vi "WILT Increment Cycle.vi"(5 "Station Number in":u32, 6 "Short Cycle?":bool, 7 "Day/Night Cycle":T7, 8 "Error In":errorcluster, 10 "Station Test State In":T1, 11 "Dryer Step 5 In":T3 {"Night Cycle Count" format="%04d"; "Day Cycle Count" format="%04d"}) -> (0 "Error Out":errorcluster, 1 "Enable Start Retry":bool, 2 "Test Station Out":T1, 3 "Dryer Step 5 Output":T3 {"Night Cycle Count" format="%04d"; "Day Cycle Count" format="%04d"})   [LabVIEW 2016]
uses:
  Type Definitions/WILT Day Night Cycle Enum.ctl
  Type Definitions/WILT Dryer.ctl
  Type Definitions/WILT Dryer Details.ctl
  Type Definitions/WILT Agilent Channel Definition.ctl
  Type Definitions/WILT DAQ Data.ctl
  Type Definitions/WILT Station Test State Cluster.ctl
  Type Definitions/WILT Dryer Test State.ctl
panel:
  # "Day"
  # "Night"
  # "Day"
  # "Night"
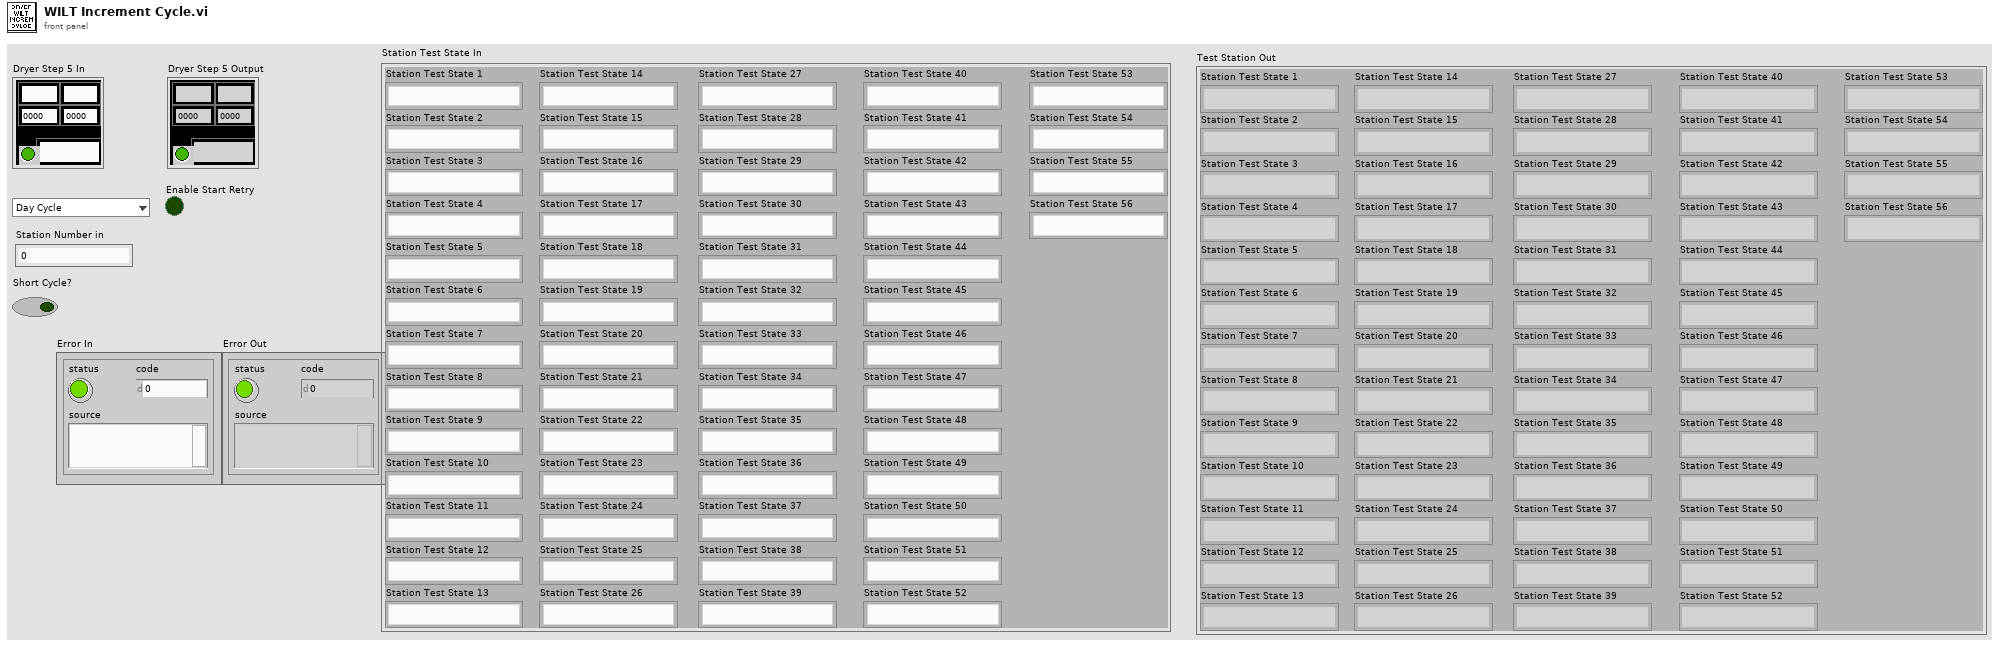
[diagram p1: front panel]
types:
  T1 = typedef "WILT Station Test State Cluster.ctl" = cluster{"Station Test State 1":T2, "Station Test State 2":T2, "Station Test State 3":T2, "Station Test State 4":T2, "Station Test State 5":T2, "Station Test State 6":T2, "Station Test State 7":T2, "Station Test State 8":T2, "Station Test State 9":T2, "Station Test State 10":T2, "Station Test State 11":T2, "Station Test State 12":T2, "Station Test State 13":T2, "Station Test State 14":T2, "Station Test State 15":T2, "Station Test State 16":T2, "Station Test State 17":T2, "Station Test State 18":T2, "Station Test State 19":T2, "Station Test State 20":T2, "Station Test State 21":T2, "Station Test State 22":T2, "Station Test State 23":T2, "Station Test State 24":T2, "Station Test State 25":T2, "Station Test State 26":T2, "Station Test State 27":T2, "Station Test State 28":T2, "Station Test State 29":T2, "Station Test State 30":T2, "Station Test State 31":T2, "Station Test State 32":T2, "Station Test State 33":T2, "Station Test State 34":T2, "Station Test State 35":T2, "Station Test State 36":T2, "Station Test State 37":T2, "Station Test State 38":T2, "Station Test State 39":T2, "Station Test State 40":T2, "Station Test State 41":T2, "Station Test State 42":T2, "Station Test State 43":T2, "Station Test State 44":T2, "Station Test State 45":T2, "Station Test State 46":T2, "Station Test State 47":T2, "Station Test State 48":T2, "Station Test State 49":T2, "Station Test State 50":T2, "Station Test State 51":T2, "Station Test State 52":T2, "Station Test State 53":T2, "Station Test State 54":T2, "Station Test State 55":T2, "Station Test State 56":T2}
  T2 = typedef "WILT Dryer Test State.ctl" = enum16{"No Serial Number", "Waiting for Dryer To Start", "Drying Clothes", "Water Injection 1 (On)", "Water Injection 1 Timer", "Water Injection 1 (Off)", "Pause Dryer", "Sending Start Stop CMD", "Pause Dryer 2", "Sending Start Stop CMD 2", "Drying Clothes 2", "Water Injection 2 (On)", "Water Injection 2 Timer", "Water Injection 2 (Off)", "Drying Clothes 3", "Cooling Down", "Sending Start Stop CMD 3", "Increment Cycle"}
  T3 = typedef "WILT Dryer.ctl" = cluster{"Lab ID":string, "Day Cycle Count":i32, "Station Label":string, "Dryer Details":T4, "Status Color":u32, "Invisible Button":bool, "Night Cycle Count":i32, "Station Index":i32, "Cycle Index":string, "Audit Alert":bool, "Agilent Channel Definition":T5, "DAQ Data":T6}
  T4 = typedef "WILT Dryer Details.ctl" = cluster{"Station":string, "Lab ID":string, "TR Number":string}
  T5 = typedef "WILT Agilent Channel Definition.ctl" = cluster{"Channel":string, "Station":string, "Label":string, "Agilent Station":string, "Data":dbl}
  T6 = typedef "WILT DAQ Data.ctl" = cluster{"L1 Current":dbl, "L2 Current":dbl, "Temperature  Deg F (TC)":dbl, "Volts":dbl, "Volts (208)":dbl, "SW (208)":dbl}
  T7 = typedef "WILT Day Night Cycle Enum.ctl" = enum16{"Day Cycle", "Night Cycle", "Day Cycle (No Water)"}
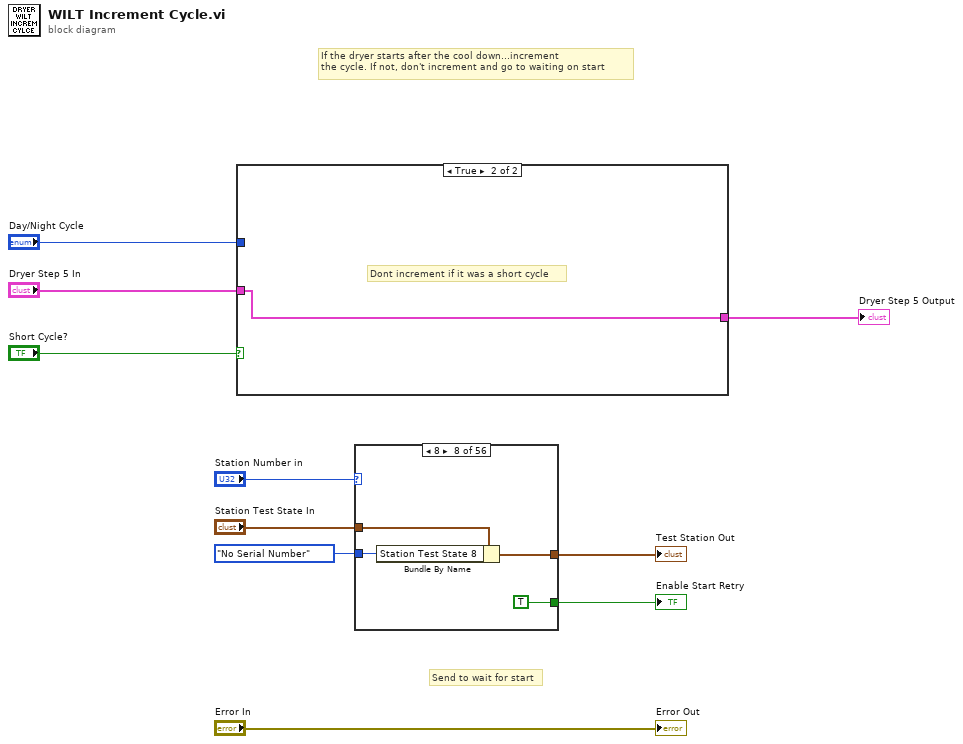
[diagram p0: block diagram]
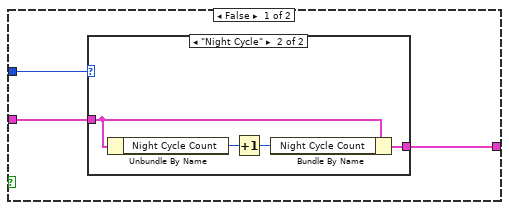
[diagram p2: hidden frame]
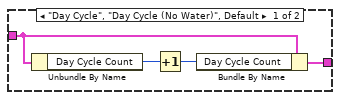
[diagram p3: hidden frame]
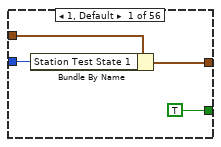
[diagram p4: hidden frame]
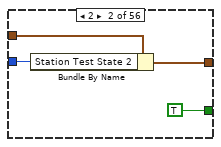
[diagram p5: hidden frame]
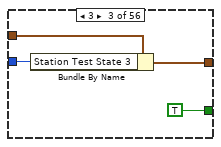
[diagram p6: hidden frame]
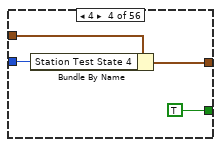
[diagram p7: hidden frame]
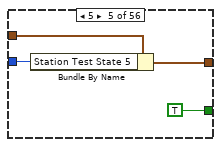
[diagram p8: hidden frame]
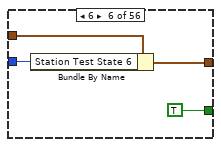
[diagram p9: hidden frame]
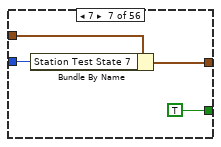
[diagram p10: hidden frame]
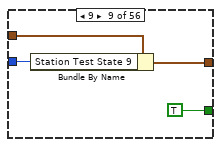
[diagram p11: hidden frame]
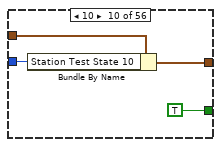
[diagram p12: hidden frame]
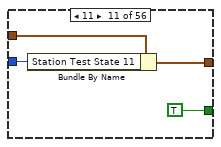
[diagram p13: hidden frame]
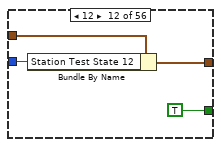
[diagram p14: hidden frame]
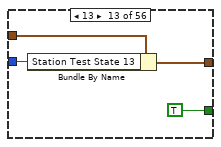
[diagram p15: hidden frame]
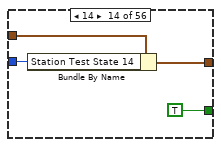
[diagram p16: hidden frame]
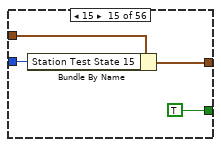
[diagram p17: hidden frame]
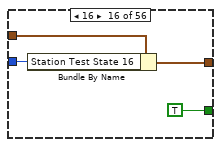
[diagram p18: hidden frame]
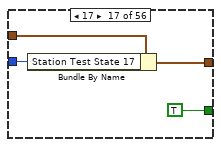
[diagram p19: hidden frame]
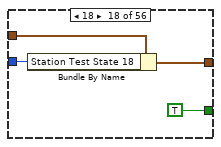
[diagram p20: hidden frame]
diagram:
  # "Send to wait for start"
  # "If the dryer starts after the cool down...increment\nthe cycle. If not, don't increment and go to waiting on start"
  n1 = case shown="True" "Short Cycle?" {
    tunnel: "Day/Night Cycle" -> [w13 _]
    tunnel: [w12 w22] -> w8
    tunnel: "Dryer Step 5 In" -> [w11 w22]
    frame False {
      n2 = case shown="\"Night Cycle\"" w13 {
        tunnel: w11 -> [w14 w18]
        tunnel: [w17 w21] -> w12
        frame "Day Cycle", "Day Cycle (No Water)", Default {
          n3 = Unbundle By Name(w14) -> ("Day Cycle Count"=w16:i32)
          n4 = Increment(x=w16) -> (x+1=w15:i32)
          n5 = Bundle By Name(cluster=w14, "Day Cycle Count"=w15) -> (w17:T3)
        }
        frame "Night Cycle" {
          n6 = Unbundle By Name(w18) -> ("Night Cycle Count"=w20:i32)
          n7 = Increment(x=w20) -> (x+1=w19:i32)
          n8 = Bundle By Name(cluster=w18, "Night Cycle Count"=w19) -> (w21:T3)
        }
      }
    }
    frame True {
      # "Dont increment if it was a short cycle"
    }
  }
  "Dryer Step 5 Output" <- w8
  n9 = case shown="8" "Station Number in" {
    tunnel: "Station Test State In" -> [w26 w30 w34 w38 w42 w46 w50 w54 w58 w62 w66 w70 w74 w78 w82 w86 w90 w94 w98 w102 w106 w110 w114 w118 w122 w126 w130 w134 w138 w142 w146 w150 w154 w158 w162 w166 w170 w174 w178 w182 w186 w190 w194 w198 w202 w206 w210 w214 w218 w222 w226 w230 w234 w238 w242 w246]
    tunnel: WILT_Dryer_Test_State."No Serial Number" ("Station Test State 56") -> [w25 w28 w32 w36 w40 w44 w48 w52 w56 w60 w64 w68 w72 w76 w80 w84 w88 w92 w96 w100 w104 w108 w112 w116 w120 w124 w128 w132 w136 w140 w144 w148 w152 w156 w160 w164 w168 w172 w176 w180 w184 w188 w192 w196 w200 w204 w208 w212 w216 w220 w224 w228 w232 w236 w240 w244]
    tunnel: [w24 w29 w33 w37 w41 w45 w49 w53 w57 w61 w65 w69 w73 w77 w81 w85 w89 w93 w97 w101 w105 w109 w113 w117 w121 w125 w129 w133 w137 w141 w145 w149 w153 w157 w161 w165 w169 w173 w177 w181 w185 w189 w193 w197 w201 w205 w209 w213 w217 w221 w225 w229 w233 w237 w241 w245] -> w5
    tunnel: [TRUE TRUE TRUE TRUE TRUE TRUE TRUE TRUE TRUE TRUE TRUE TRUE TRUE TRUE TRUE TRUE TRUE TRUE TRUE TRUE TRUE TRUE TRUE TRUE TRUE TRUE TRUE TRUE TRUE TRUE TRUE TRUE TRUE TRUE TRUE TRUE TRUE TRUE TRUE TRUE TRUE TRUE TRUE TRUE TRUE TRUE TRUE TRUE TRUE TRUE TRUE TRUE TRUE TRUE TRUE TRUE] -> w2
    frame 1, Default {
      n10 = Bundle By Name(cluster=w26, "Station Test State 1"=w25) -> (w24:T1)
    }
    frame 2 {
      n11 = Bundle By Name(cluster=w30, "Station Test State 2"=w28) -> (w29:T1)
    }
    frame 3 {
      n12 = Bundle By Name(cluster=w34, "Station Test State 3"=w32) -> (w33:T1)
    }
    frame 4 {
      n13 = Bundle By Name(cluster=w38, "Station Test State 4"=w36) -> (w37:T1)
    }
    frame 5 {
      n14 = Bundle By Name(cluster=w42, "Station Test State 5"=w40) -> (w41:T1)
    }
    frame 6 {
      n15 = Bundle By Name(cluster=w46, "Station Test State 6"=w44) -> (w45:T1)
    }
    frame 7 {
      n16 = Bundle By Name(cluster=w50, "Station Test State 7"=w48) -> (w49:T1)
    }
    frame 8 {
      n17 = Bundle By Name(cluster=w54, "Station Test State 8"=w52) -> (w53:T1)
    }
    frame 9 {
      n18 = Bundle By Name(cluster=w58, "Station Test State 9"=w56) -> (w57:T1)
    }
    frame 10 {
      n19 = Bundle By Name(cluster=w62, "Station Test State 10"=w60) -> (w61:T1)
    }
    frame 11 {
      n20 = Bundle By Name(cluster=w66, "Station Test State 11"=w64) -> (w65:T1)
    }
    frame 12 {
      n21 = Bundle By Name(cluster=w70, "Station Test State 12"=w68) -> (w69:T1)
    }
    frame 13 {
      n22 = Bundle By Name(cluster=w74, "Station Test State 13"=w72) -> (w73:T1)
    }
    frame 14 {
      n23 = Bundle By Name(cluster=w78, "Station Test State 14"=w76) -> (w77:T1)
    }
    frame 15 {
      n24 = Bundle By Name(cluster=w82, "Station Test State 15"=w80) -> (w81:T1)
    }
    frame 16 {
      n25 = Bundle By Name(cluster=w86, "Station Test State 16"=w84) -> (w85:T1)
    }
    frame 17 {
      n26 = Bundle By Name(cluster=w90, "Station Test State 17"=w88) -> (w89:T1)
    }
    frame 18 {
      n27 = Bundle By Name(cluster=w94, "Station Test State 18"=w92) -> (w93:T1)
    }
    frame 19 {
      n28 = Bundle By Name(cluster=w98, "Station Test State 19"=w96) -> (w97:T1)
    }
    frame 20 {
      n29 = Bundle By Name(cluster=w102, "Station Test State 20"=w100) -> (w101:T1)
    }
    frame 21 {
      n30 = Bundle By Name(cluster=w106, "Station Test State 21"=w104) -> (w105:T1)
    }
    frame 22 {
      n31 = Bundle By Name(cluster=w110, "Station Test State 22"=w108) -> (w109:T1)
    }
    frame 23 {
      n32 = Bundle By Name(cluster=w114, "Station Test State 23"=w112) -> (w113:T1)
    }
    frame 24 {
      n33 = Bundle By Name(cluster=w118, "Station Test State 24"=w116) -> (w117:T1)
    }
    frame 25 {
      n34 = Bundle By Name(cluster=w122, "Station Test State 25"=w120) -> (w121:T1)
    }
    frame 26 {
      n35 = Bundle By Name(cluster=w126, "Station Test State 26"=w124) -> (w125:T1)
    }
    frame 27 {
      n36 = Bundle By Name(cluster=w130, "Station Test State 27"=w128) -> (w129:T1)
    }
    frame 28 {
      n37 = Bundle By Name(cluster=w134, "Station Test State 28"=w132) -> (w133:T1)
    }
    frame 29 {
      n38 = Bundle By Name(cluster=w138, "Station Test State 29"=w136) -> (w137:T1)
    }
    frame 30 {
      n39 = Bundle By Name(cluster=w142, "Station Test State 30"=w140) -> (w141:T1)
    }
    frame 31 {
      n40 = Bundle By Name(cluster=w146, "Station Test State 31"=w144) -> (w145:T1)
    }
    frame 32 {
      n41 = Bundle By Name(cluster=w150, "Station Test State 32"=w148) -> (w149:T1)
    }
    frame 33 {
      n42 = Bundle By Name(cluster=w154, "Station Test State 33"=w152) -> (w153:T1)
    }
    frame 34 {
      n43 = Bundle By Name(cluster=w158, "Station Test State 34"=w156) -> (w157:T1)
    }
    frame 35 {
      n44 = Bundle By Name(cluster=w162, "Station Test State 35"=w160) -> (w161:T1)
    }
    frame 36 {
      n45 = Bundle By Name(cluster=w166, "Station Test State 36"=w164) -> (w165:T1)
    }
    frame 37 {
      n46 = Bundle By Name(cluster=w170, "Station Test State 37"=w168) -> (w169:T1)
    }
    frame 38 {
      n47 = Bundle By Name(cluster=w174, "Station Test State 38"=w172) -> (w173:T1)
    }
    frame 39 {
      n48 = Bundle By Name(cluster=w178, "Station Test State 39"=w176) -> (w177:T1)
    }
    frame 40 {
      n49 = Bundle By Name(cluster=w182, "Station Test State 40"=w180) -> (w181:T1)
    }
    frame 41 {
      n50 = Bundle By Name(cluster=w186, "Station Test State 41"=w184) -> (w185:T1)
    }
    frame 42 {
      n51 = Bundle By Name(cluster=w190, "Station Test State 42"=w188) -> (w189:T1)
    }
    frame 43 {
      n52 = Bundle By Name(cluster=w194, "Station Test State 43"=w192) -> (w193:T1)
    }
    frame 44 {
      n53 = Bundle By Name(cluster=w198, "Station Test State 44"=w196) -> (w197:T1)
    }
    frame 45 {
      n54 = Bundle By Name(cluster=w202, "Station Test State 45"=w200) -> (w201:T1)
    }
    frame 46 {
      n55 = Bundle By Name(cluster=w206, "Station Test State 46"=w204) -> (w205:T1)
    }
    frame 47 {
      n56 = Bundle By Name(cluster=w210, "Station Test State 47"=w208) -> (w209:T1)
    }
    frame 48 {
      n57 = Bundle By Name(cluster=w214, "Station Test State 48"=w212) -> (w213:T1)
    }
    frame 49 {
      n58 = Bundle By Name(cluster=w218, "Station Test State 49"=w216) -> (w217:T1)
    }
    frame 50 {
      n59 = Bundle By Name(cluster=w222, "Station Test State 50"=w220) -> (w221:T1)
    }
    frame 51 {
      n60 = Bundle By Name(cluster=w226, "Station Test State 51"=w224) -> (w225:T1)
    }
    frame 52 {
      n61 = Bundle By Name(cluster=w230, "Station Test State 52"=w228) -> (w229:T1)
    }
    frame 53 {
      n62 = Bundle By Name(cluster=w234, "Station Test State 53"=w232) -> (w233:T1)
    }
    frame 54 {
      n63 = Bundle By Name(cluster=w238, "Station Test State 54"=w236) -> (w237:T1)
    }
    frame 55 {
      n64 = Bundle By Name(cluster=w242, "Station Test State 55"=w240) -> (w241:T1)
    }
    frame 56 {
      n65 = Bundle By Name(cluster=w246, "Station Test State 56"=w244) -> (w245:T1)
    }
  }
  "Test Station Out" <- w5
  "Enable Start Retry" <- w2
  "Error Out" <- "Error In"
